vi "Create Pattern.vi"(0 "Vector Statements":string[](array[string]), 1 "Name":string, 11 "error in (no error)":errorcluster) -> (4 "Digital Pattern":string, 15 "error out":errorcluster)   [LabVIEW 2018, in "MIPI RFFE API.lvlib"]
uses:
  MIPI RFFE API.lvlib
  <vilib>/Utility/error.llb/whitespace.ctl
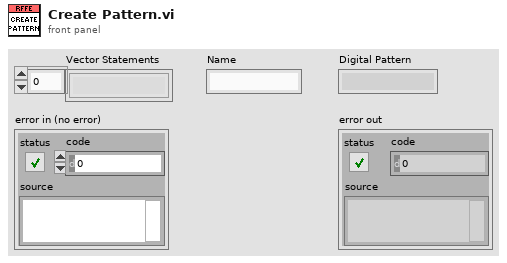
[diagram p1: front panel]
types:
  T1 = typedef "whitespace.ctl" = u16
  T2 = cluster{"Major":u16, "Minor":u16, "Fix":u16, "Build":u16}
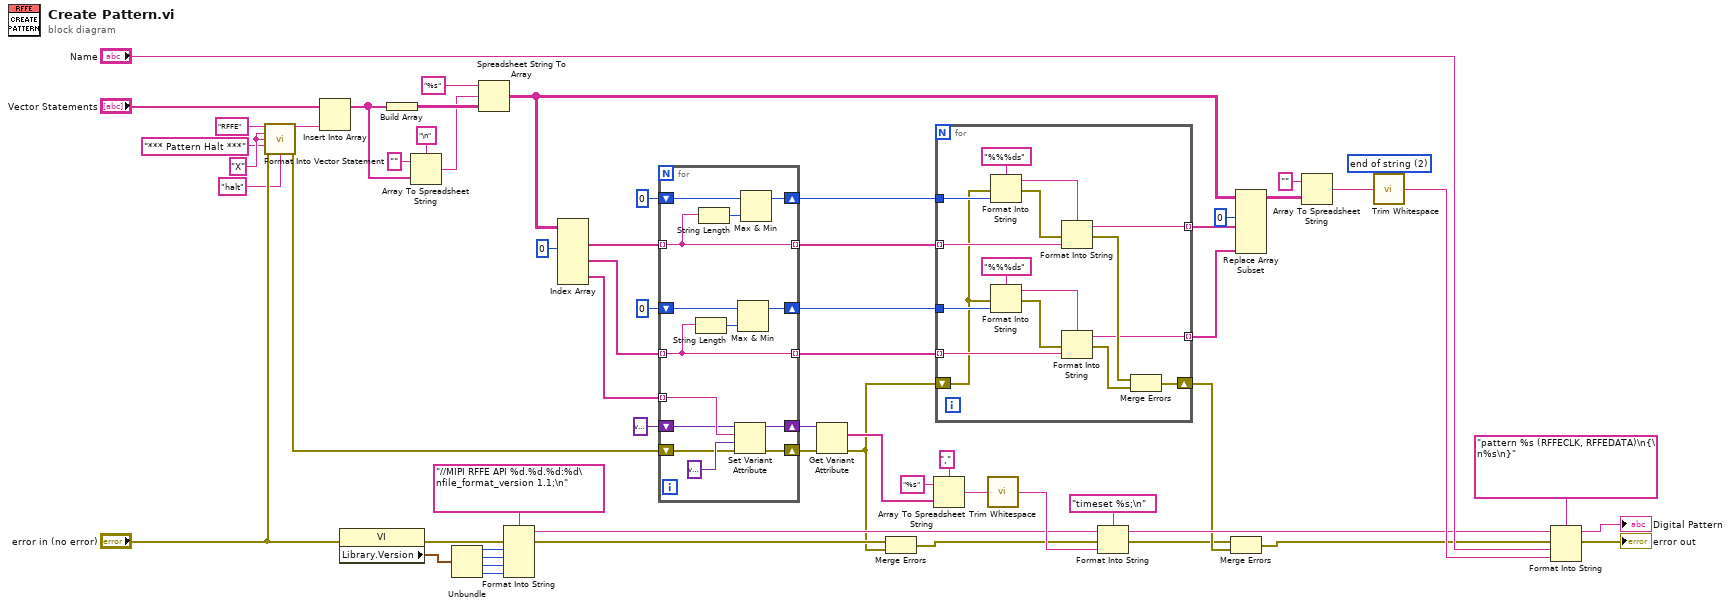
[diagram p0: block diagram]
diagram:
  w22 = T1 2 items=["both", "start of string", "end of string"] ("location (both)")
  w45 = "X" ("CLK")
  n1 = call "Format Into Vector Statement.vi"("Timeset (RFFE)"="RFFE" ("Timeset"), "CLK (1)"=w45, "DATA (0)"=w45, "Comment"="*** Pattern Halt ***", "error in (no error)"="error in (no error)", "Opcode"="halt") -> ("Vector Statement"=w43:string, "error out"=w44:errorcluster)  [unwired: 8 in]
  n2 = Insert Into Array(array="Vector Statements", new element=w43) -> (w41:string[])  [unwired: 1 in]
  n3 = property class="VI"(error in="error in (no error)") -> (error out=w19:errorcluster, "Library.Version"=w21:T2)  [unwired: 1 in, 1 out]
  n4 = Build Array(w41) -> (w58:string[][])
  n5 = Array To Spreadsheet String(delimiter (Tab)="\n", array=w41, 3:"" ("format string")) -> (spreadsheet string=w48:string)
  n6 = Unbundle(w21) -> ("Major"=w20:u16, "Minor"=w13:u16, "Fix"=w12:u16, "Build"=w11:u16)
  n7 = Spreadsheet String To Array(format string="%s", spreadsheet string=w48, array type (2D Dbl)=w58) -> (array=w30:string[][])  [unwired: 1 in]
  n8 = Format Into String(format string="//MIPI RFFE API %d.%d.%d:%d\nfile_format_version 1.1;\n", error in=w19, w20, w13, w12, w11) -> (resulting string=w9:string, error out=w6:errorcluster)  [unwired: 1 in]
  n9 = Index Array(array=w30, index (col) #1=0 ("disabled index (col)")) -> (element #1=w38:string[], element #2=w39:string[], element #3=w40:string[])  [unwired: 5 in]
  n10 = for {
    tunnel: w40 -> [w75] mode=indexing
    shift-right: [w72] -> w55
    shift-left: variant ("variant") -> [w74]
    shift-right: [w71] -> w51
    shift-left: w44 -> [w70]
    tunnel: w39 -> [w62] mode=indexing
    tunnel: w38 -> [w63] mode=indexing
    shift-right: [w68] -> w31
    shift-left: 0 ("length") -> [w69]
    shift-right: [w64] -> w32
    shift-left: 0 ("length") -> [w65]
    tunnel: [w63] -> w34 mode=indexing
    tunnel: [w62] -> w33 mode=indexing
    n11 = String Length(string=w62) -> (length=w67:i32)
    n12 = String Length(string=w63) -> (length=w66:i32)
    n13 = Set Variant Attribute(Variant=w74, name=w75, value=variant, error in=w70) -> (Variant out=w72:variant, error out=w71:errorcluster)  [unwired: 1 out]
    n14 = Max & Min(x=w69, y=w67) -> (max(x,y)=w68:i32)  [unwired: 1 out]
    n15 = Max & Min(x=w65, y=w66) -> (max(x,y)=w64:i32)  [unwired: 1 out]
  }
  n16 = Get Variant Attribute(Variant=w55, error in=w51) -> (names=w54:string[], error out=w5:errorcluster)  [unwired: 2 in, 2 out]
  n17 = Merge Errors(w6, w5) -> (w4:errorcluster)
  n18 = Array To Spreadsheet String(delimiter (Tab)=",", array=w54, 3:"%s" ("format string")) -> (spreadsheet string=w50:string)
  n19 = for {
    tunnel: w34 -> [w89] mode=indexing
    tunnel: w33 -> [w84] mode=indexing
    shift-right: [w78] -> w3
    shift-left: w5 -> [w83]
    tunnel: w32 -> [w90]
    tunnel: w31 -> [w85]
    tunnel: [w77] -> w29 mode=indexing
    tunnel: [w76] -> w28 mode=indexing
    n20 = Format Into String(format string="%%%ds", error in=w83, w90) -> (resulting string=w88:string, error out=w82:errorcluster)  [unwired: 1 in]
    n21 = Format Into String(format string="%%%ds", error in=w83, w85) -> (resulting string=w87:string, error out=w81:errorcluster)  [unwired: 1 in]
    n22 = Format Into String(format string=w88, error in=w82, w89) -> (resulting string=w77:string, error out=w80:errorcluster)  [unwired: 1 in]
    n23 = Format Into String(format string=w87, error in=w81, w84) -> (resulting string=w76:string, error out=w79:errorcluster)  [unwired: 1 in]
    n24 = Merge Errors(w80, w79) -> (w78:errorcluster)
  }
  n25 = call <vilib>:"Trim Whitespace.vi"("string"=w50) -> ("trimmed string"=w14:string)  [unwired: 1 in]
  n26 = Format Into String(format string="timeset %s;\n", initial string=w9, error in=w4, w14) -> (resulting string=w8:string, error out=w2:errorcluster)
  n27 = Merge Errors(w2, w3) -> (w1:errorcluster)
  n28 = Replace Array Subset(array=w30, new element #1=w29, index (col) #1=0 ("disabled index (col)"), new element #2=w28) -> (w27:string[][])  [unwired: 3 in]
  n29 = Array To Spreadsheet String(array=w27, 3:"" ("format string")) -> (spreadsheet string=w23:string)  [unwired: 1 in]
  n30 = call <vilib>:"Trim Whitespace.vi"("string"=w23, "location (both)"=w22) -> ("trimmed string"=w10:string)
  n31 = Format Into String(format string="pattern %s (RFFECLK, RFFEDATA)\n{\n%s\n}", initial string=w8, error in=w1, "Name", w10) -> (resulting string=→"Digital Pattern":string, error out=→"error out":errorcluster)
